vi "Run VI.vi"(4 "Indicator Names":string[](array[string]), 6 "Open Front Panel":bool=TRUE, 7 "Run Options":i32, 8 "error in (no error)":errorcluster, 9 "VI Control Values":refnum<class "tBSONDocument.lvclass">, 10 "VI Path":string, 11 "tWorkerCommandRunner in":refnum<class "tWorkerCommandRunner.lvclass">) -> (0 "error out":errorcluster, 3 "tWorkerCommandRunner out":refnum<class "tWorkerCommandRunner.lvclass">)   [LabVIEW 2014, in "tWorkerCommandRunner.lvlib" / "tWorkerCommandRunner.lvclass"]
uses:
  tWorkerCommandRunner.lvclass
  BSON/tBSONDocument/tBSONDocument.lvclass
  <vilib>/ActorFramework/Actor/Actor.lvclass/Actor.ctl
  BSON/tBSONElement/tBSONElement.lvclass
  tWorkerTCPConnection/msgs/Return Run VI State Msg/Return Run VI State Msg.lvclass
  <vilib>/ActorFramework/Actor/Actor.lvclass
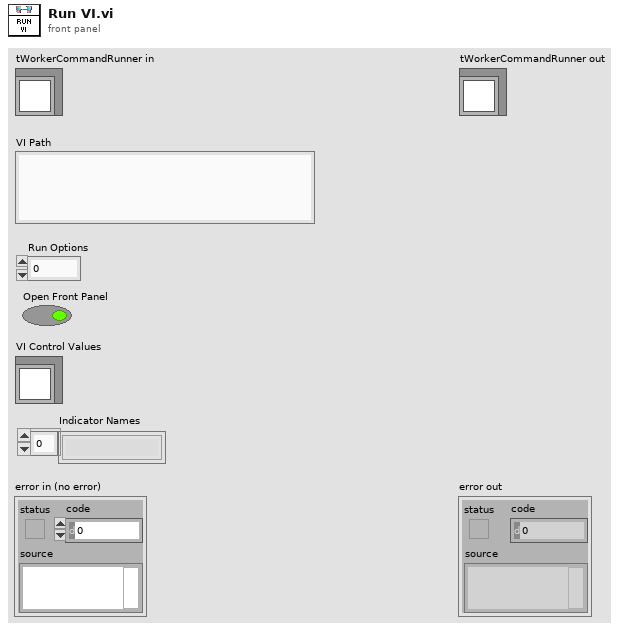
[diagram p1: front panel]
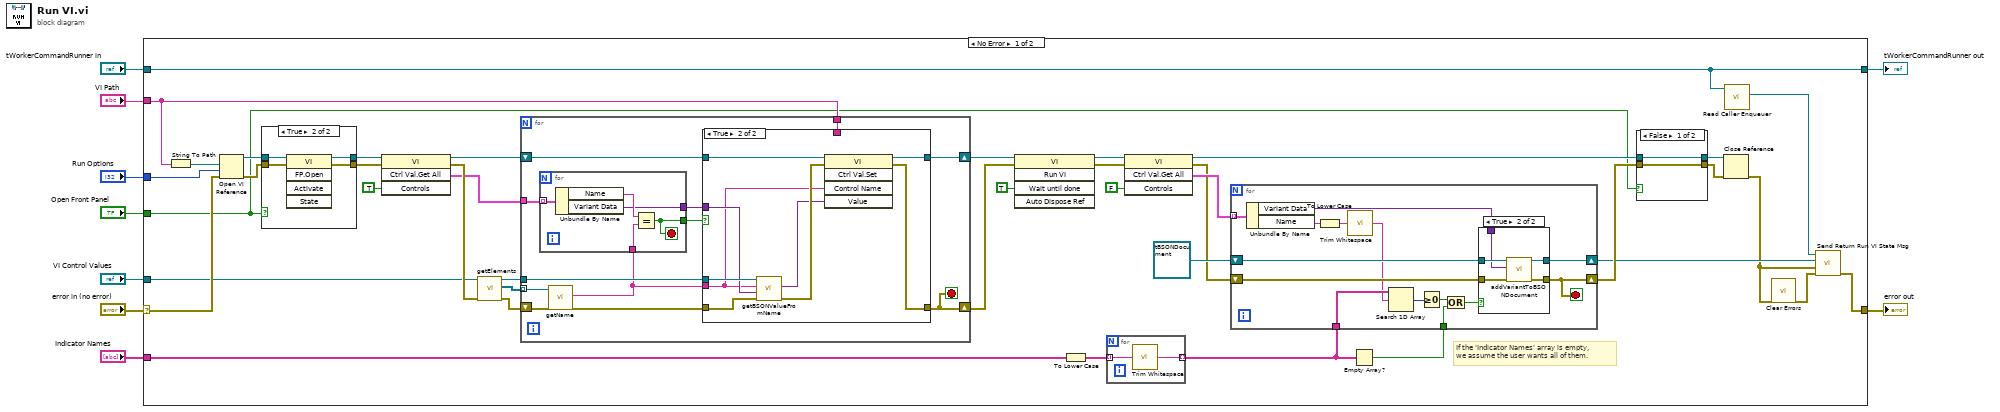
[diagram p0: block diagram]
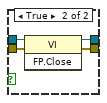
[diagram p2: hidden frame]
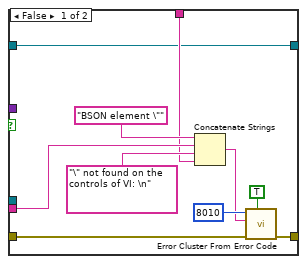
[diagram p5: hidden frame]
diagram:
  n1 = case shown="No Error" "error in (no error)" {
    selector: "error in (no error)" -> [w48 w122]
    tunnel: [w17 w122] -> w8
    tunnel: [w19 w121] -> w6
    tunnel: "tWorkerCommandRunner in" -> [w19 w121]
    tunnel: "VI Path" -> [w34 _]
    tunnel: "Run Options" -> [w47 _]
    tunnel: "VI Control Values" -> [w40 _]
    tunnel: "Open Front Panel" -> [w14 _]
    tunnel: "Indicator Names" -> [w12 _]
    frame No Error {
      # "If the 'Indicator Names' array is empty,\nwe assume the user wants all of them."
      n2 = String To Path(string=w34) -> (path=w49:path)
      n3 = Open VI Reference(vi path=w49, options=w47, error in (no error)=w48) -> (vi reference=w46:refnum<vi>, error out=w45:errorcluster)  [unwired: 3 in]
      n4 = case shown="True" w14 {
        tunnel: w46 -> [w59 w63]
        tunnel: w45 -> [w58 w62]
        tunnel: [w59 w61] -> w44
        tunnel: [w58 w60] -> w43
        frame False {
        }
        frame True {
          n5 = invoke class="VI" method="FP.Open"(reference=w63, error in=w62) -> (reference out=w61:refnum<vi>, error out=w60:errorcluster)  [unwired: 3 in, 3 out]
        }
      }
      n6 = invoke class="VI" method="Ctrl Val.Get All"(reference=w44, error in=w43, "Controls"=TRUE) -> (reference out=w35:refnum<vi>, error out=w41:errorcluster, "Get All Control Values Variant"=w37:cluster{"Name":string, "Variant Data":variant}[])  [unwired: 1 in, 1 out]
      n7 = call "getElements.vi"("error in (no error)"=w41, "tBSONDocument in"=w40) -> ("error out"=w39:errorcluster, "Elements"=w38:refnum<class "tBSONElement.lvclass">[], "tBSONDocument out"=w36:refnum<class "tBSONDocument.lvclass">)  [unwired: 7 in]
      n8 = for {
        tunnel: w38 -> [w96] mode=indexing
        shift-right: [w85] -> w32
        shift-left: w39 -> [w95]
        tunnel: w37 -> [w94]
        tunnel: w36 -> [w92]
        shift-right: [w86] -> w33
        shift-left: w35 -> [w89]
        tunnel: w34 -> [w87]
        stop <- w85 stop-if-true
        n9 = call "getName.vi"("error in (no error)"=w95, "tBSONElement in"=w96) -> ("error out"=w93:errorcluster, "Name"=w88:string)  [unwired: 7 in, 1 out]
        n10 = for {
          tunnel: w94 -> [w120] mode=indexing
          tunnel: w88 -> [w118]
          tunnel: [w117] -> w90
          tunnel: [w116] -> w91
          stop <- w116 stop-if-true
          n11 = Unbundle By Name(w120) -> ("Name"=w119:string, "Variant Data"=w117:variant)
          n12 = Equal?(x=w119, y=w118) -> (x = y?=w116:bool)
        }
        n13 = case shown="True" w91 {
          tunnel: w93 -> [w106 w114]
          tunnel: w92 -> [_ w115]
          tunnel: w90 -> [_ w113]
          tunnel: w89 -> [w97 w112]
          tunnel: w88 -> [w100 w110]
          tunnel: [w103 w107] -> w85
          tunnel: w87 -> [w98 _]
          tunnel: [w97 w108] -> w86
          frame False {
            n14 = Concatenate Strings("BSON element \"" ("string"), w100, "\" not found on the controls of VI: \n" ("string"), w98) -> (w101:string)
            n15 = call <vilib>:"Error Cluster From Error Code.vi"("show call chain? (False)"=TRUE, "error in (no error)"=w106, "error message (\"\")"=w101, "error code (0)"=8010) -> ("error out"=w103:errorcluster)  [unwired: 5 in]
          }
          frame True {
            n16 = call "getBSONValueFromName.vi"("error in (no error)"=w114, "Cluster Type (optional)"=w113, "Element Name"=w110, "tBSONDocument in"=w115) -> ("error out"=w111:errorcluster, "Variant"=w109:variant)  [unwired: 5 in, 1 out]
            n17 = invoke class="VI" method="Ctrl Val.Set"(reference=w112, error in=w111, "Control Name"=w110, "Value"=w109) -> (reference out=w108:refnum<vi>, error out=w107:errorcluster)  [unwired: 1 in, 3 out]
          }
        }
      }
      n18 = invoke class="VI" method="Run VI"(reference=w33, error in=w32, "Wait until done"=TRUE ("Wait Until Done")) -> (reference out=w30:refnum<vi>, error out=w29:errorcluster)  [unwired: 2 in, 3 out]
      n19 = To Lower Case(string=w12) -> (all lower case string=w11:string[])
      n20 = for {
        tunnel: w11 -> [w51] mode=indexing
        tunnel: [w50] -> w10 mode=indexing
        n21 = call <vilib>:"Trim Whitespace.vi"("string"=w51) -> ("trimmed string"=w50:string)  [unwired: 1 in]
      }
      n22 = invoke class="VI" method="Ctrl Val.Get All"(reference=w30, error in=w29, "Controls"=FALSE) -> (reference out=w24:refnum<vi>, error out=w25:errorcluster, "Get All Control Values Variant"=w27:cluster{"Name":string, "Variant Data":variant}[])  [unwired: 1 in, 1 out]
      n23 = Empty Array?(array=w10) -> (empty?=w13:bool)
      n24 = for {
        tunnel: w27 -> [w75] mode=indexing
        shift-right: [w76] -> w20
        shift-left: refnum<class "tBSONDocument.lvclass"> refnum ("tBSONDocument in") -> [w77]
        shift-right: [w67] -> w23
        shift-left: w25 -> [w74]
        tunnel: w10 -> [w72]
        tunnel: w13 -> [w69]
        stop <- w67 stop-if-true
        n25 = Unbundle By Name(w75) -> ("Variant Data"=w73:variant, "Name"=w66:string)
        n26 = To Lower Case(string=w66) -> (all lower case string=w65:string)
        n27 = call <vilib>:"Trim Whitespace.vi"("string"=w65) -> ("trimmed string"=w64:string)  [unwired: 1 in]
        n28 = Search 1D Array(1D array=w72, element=w64) -> (index of element=w71:i32)  [unwired: 1 in]
        n29 = Greater Or Equal To 0?(x=w71) -> (x >= 0?=w70:bool)
        n30 = Or(x=w70, y=w69) -> (x .or. y?=w68:bool)
        n31 = case shown="True" w68 {
          tunnel: w77 -> [w79 w84]
          tunnel: [w79 w83] -> w76
          tunnel: w74 -> [w78 w82]
          tunnel: w73 -> [_ w81]
          tunnel: [w78 w80] -> w67
          frame False {
          }
          frame True {
            n32 = call "addVariantToBSONDocument.vi"("error in (no error)"=w82, "Variant"=w81, "tBSONDocument in"=w84) -> ("error out"=w80:errorcluster, "tBSONDocument out"=w83:refnum<class "tBSONDocument.lvclass">)  [unwired: 7 in]
          }
        }
      }
      n33 = case shown="False" w14 {
        tunnel: w24 -> [w53 w57]
        tunnel: w23 -> [w52 w56]
        tunnel: [w52 w55] -> w22
        tunnel: [w53 w54] -> w21
        frame False {
        }
        frame True {
          n34 = invoke class="VI" method="FP.Close"(reference=w57, error in=w56) -> (reference out=w54:refnum<vi>, error out=w55:errorcluster)  [unwired: 1 in, 1 out]
        }
      }
      n35 = Close Reference(reference=w21, error in (no error)=w22) -> (error out=w16:errorcluster)
      n36 = call <vilib>:"Read Caller Enqueuer.vi"("Actor"=w19) -> ("Caller Enqueuer"=w18:refnum<class "Message Enqueuer.lvclass">)  [unwired: 10 in]
      n37 = call <vilib>:"Clear Errors.vi"("error in (no error)"=w16) -> ("error out"=w15:errorcluster)  [unwired: 5 in, 1 out]
      n38 = call "Send Return Run VI State Msg.vi"("error in (no error)"=w15, "Error From Run VI"=w16, "Indicators"=w20, "Message Enqueuer"=w18) -> ("error out"=w17:errorcluster)  [unwired: 6 in, 1 out]
    }
    frame Error {
    }
  }
  "error out" <- w8
  "tWorkerCommandRunner out" <- w6
